vi "ReadAllChnlParams.vi"(8 "error in (no error)":errorcluster, 10 "ChnlName":string, 11 "BME_DG_System in":refnum<class "BME_DG_System.lvclass">) -> (0 "error out":errorcluster, 1 "Name of Card":string, 2 "ChnlParam":T1={"Channel Name"="", "ChnParameter"={" Delay (µs)"=0.0, "On?"=FALSE, "PositiveVoltage?"=TRUE, "50OhmTerminated? "=FALSE, "25OhmOutput?"=FALSE}, "DelayFormula"="", "OutputModulo"=1, "Go and Done Signal"={"Go Signal"=16, "Done Signal"=16}, "G08_Chnl_Settings"={"Pulse Width (µs)"=0.1, "Output Offset"=0, "Disconnect (E,F)"=FALSE, "Onto MsBus (E,F)"=FALSE, "Input Positive (E,F)"=TRUE, "Param Change"=FALSE, "Inhibit internal clock"=FALSE}} {"ChnParameter"."Delay (µs)" min=0.0 max=100000000.0 format="%.4f"; "G08_Chnl_Settings"."Pulse Width (µs)" min=0.0 max=8947840.0 format="%#.6f"; "Go and Done Signal"."Done Signal" format="%04x" items=["Local Primary"=1, "Local Secondary"=2, "Local Force"=4, "Master Primary"=16]; "Go and Done Signal"."Go Signal" format="%04x" items=["Local Primary0x1"=1, "Local Secondary0x2"=2, "Local Force 0x4"=4, "Resynchronize 0x8"=8, "Master Prim. 0x10"=16, "Master Sec. 0x20"=32, "Master Force  0x40"=64, "System Clock 0x80"=128, "Delay Clock 0x100"=256, "Inhibit Local 0x200"=512, "Start Local 0x400"=1024, "Start Bus 0x800"=2048, "Step Back Local 0x1000"=4096, "Step Back Bus 0x2000"=8192, "RunCircle 0x4000"=16384, "SyncReload 0x8000"=32768, "From E 0x10000"=65536, "From F 0x20000"=131072, "From Bus 0x40000"=262144]}, 3 "BME_DG_System out":refnum<class "BME_DG_System.lvclass">)   [LabVIEW 2009, in "POLARIS BME DG.lvlib" / "BME_DG_System.lvclass"]
uses:
  BME_DG_System.lvclass
  Chnl Settings Complete.ctl
  LV-BME Interface/ChnlSettings.ctl
  Go_Done_Chnl_Settings.ctl
  MSBus.ctl
  SG08_Chnl_Settings.ctl
  BME_DG_G08_Chnl/BME_DG_G08_Chnl.lvclass
  BME_DG_G05P2_Chnl/BME_DG_G05P2_Chnl.lvclass
  BME_DG_Chnl/BME_DG_Chnl.lvclass
  POLARIS BME DG.lvlib
  BME_DG_Base/BME_DG_Base.lvclass
panel:
  in  "ChnlParam 2":T1 {"ChnParameter"."Delay (µs)" min=0.0 max=100000000.0 format="%.4f"; "G08_Chnl_Settings"."Pulse Width (µs)" min=0.0 max=8947840.0 format="%#.6f"; "Go and Done Signal"."Done Signal" format="%04x" items=["Local Primary"=1, "Local Secondary"=2, "Local Force"=4, "Master Primary"=16]; "Go and Done Signal"."Go Signal" format="%04x" items=["Local Primary0x1"=1, "Local Secondary0x2"=2, "Local Force 0x4"=4, "Resynchronize 0x8"=8, "Master Prim. 0x10"=16, "Master Sec. 0x20"=32, "Master Force  0x40"=64, "System Clock 0x80"=128, "Delay Clock 0x100"=256, "Inhibit Local 0x200"=512, "Start Local 0x400"=1024, "Start Bus 0x800"=2048, "Step Back Local 0x1000"=4096, "Step Back Bus 0x2000"=8192, "RunCircle 0x4000"=16384, "SyncReload 0x8000"=32768, "From E 0x10000"=65536, "From F 0x20000"=131072, "From Bus 0x40000"=262144]}
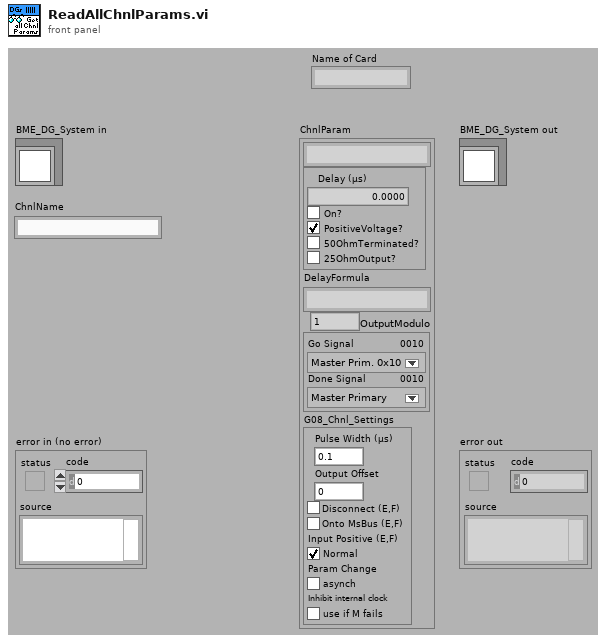
[diagram p1: front panel]
types:
  T1 = typedef "POLARIS BME DG.lvlib/Chnl Settings Complete.ctl" = cluster{"Channel Name":string, "ChnParameter":T2, "DelayFormula":string, "OutputModulo":i32, "Go and Done Signal":T3, "G08_Chnl_Settings":T5}
  T2 = typedef "POLARIS BME DG.lvlib/ChnlSettings.ctl" = cluster{" Delay (µs)":dbl, "On?":bool, "PositiveVoltage?":bool, "50OhmTerminated? ":bool, "25OhmOutput?":bool}
  T3 = typedef "POLARIS BME DG.lvlib/Go_Done_Chnl_Settings.ctl" = cluster{"Go Signal":T4, "Done Signal":u32}
  T4 = typedef "POLARIS BME DG.lvlib/MSBus.ctl" = u32
  T5 = typedef "POLARIS BME DG.lvlib/SG08_Chnl_Settings.ctl" = cluster{"Pulse Width (µs)":dbl, "Output Offset":u32, "Disconnect (E,F)":bool, "Onto MsBus (E,F)":bool, "Input Positive (E,F)":bool, "Param Change":bool, "Inhibit internal clock":bool}
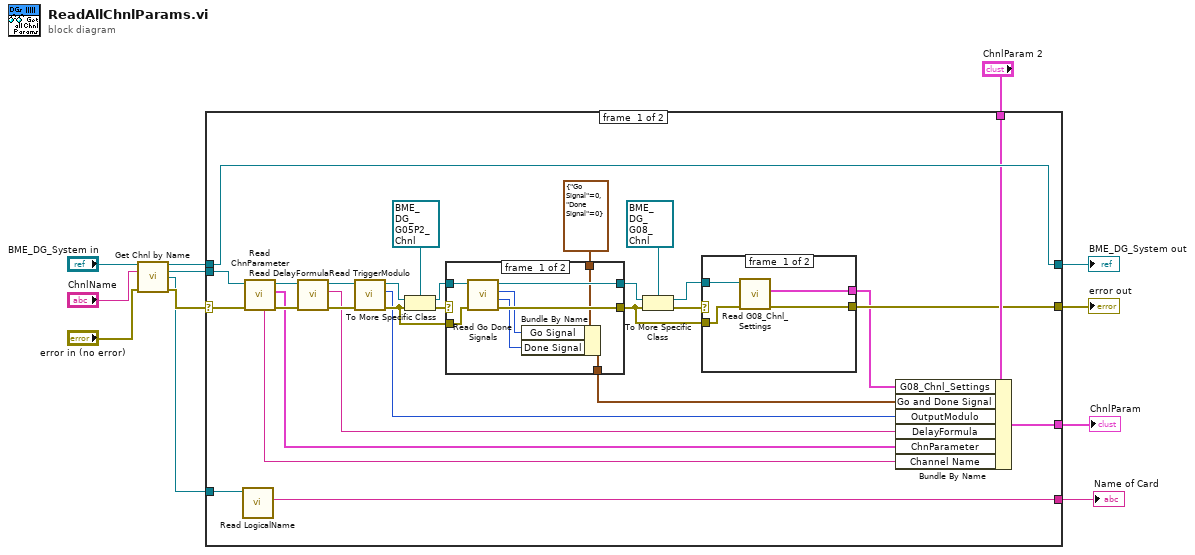
[diagram p0: block diagram]
diagram:
  n1 = call "Get Chnl by Name.vi"("BME_DG_System in"="BME_DG_System in", "Chnl Name"="ChnlName", "error in (no error)"="error in (no error)") -> ("BME_DG_System out"=w9:refnum<class "BME_DG_System.lvclass">, "BME_DG_Chnl"=w6:refnum<class "BME_DG_Chnl.lvclass">, "Owner DG"=w2:refnum<class "BME_DG_Base.lvclass">, "error out"=w7:errorcluster)  [unwired: 7 in, 2 out]
  n2 = case shown="No Error" w7 {
    selector: w7 -> [w38 w60]
    tunnel: [w23 w60] -> w12
    tunnel: [w41 w59] -> w11
    tunnel: w9 -> [w41 w59]
    tunnel: w6 -> [w39 _]
    tunnel: "ChnlParam 2" -> [w40 w58]
    tunnel: [w33 w58] -> w4
    tunnel: w2 -> [w14 _]
    tunnel: [w13 _] -> w1
    frame #0 {
      n3 = call "Read LogicalName.vi"("BME_DG_Base in"=w14) -> ("LogicalName"=w13:string)  [unwired: 8 in, 2 out]
      n4 = call-dynamic "Read ChnParameter.vi"("error in (no error)"=w38, "BME_DG_Chnl in"=w39) -> ("error out"=w36:errorcluster, "ChnParemater"=w18:T2, "BME_DG_Chnl out"=w37:refnum<class "BME_DG_Chnl.lvclass">, "Name"=w15:string)  [unwired: 4 in, 2 out]
      n5 = call-dynamic "Read DelayFormula.vi"("error in (no error)"=w36, "BME_DG_Chnl in"=w37) -> ("error out"=w34:errorcluster, "DelayFormula"=w17:string, "BME_DG_Chnl out"=w35:refnum<class "BME_DG_Chnl.lvclass">)  [unwired: 7 in]
      n6 = call-dynamic "Read TriggerModulo.vi"("error in (no error)"=w34, "BME_DG_Chnl in"=w35) -> ("error out"=w28:errorcluster, "TriggerModulo"=w16:i32, "BME_DG_Chnl out"=w32:refnum<class "BME_DG_Chnl.lvclass">)  [unwired: 7 in]
      n7 = To More Specific Class(target class=refnum<class "BME_DG_G05P2_Chnl.lvclass"> refnum ("POLARIS BME DG.lvlib:BME_DG_G05P2_Chnl.lvclass"), reference=w32, error in=w28) -> (specific class reference=w30:refnum<class "BME_DG_G05P2_Chnl.lvclass">, error out=w29:errorcluster)
      n8 = case shown="No Error" w29 {
        tunnel: w30 -> [w54 w56]
        tunnel: [w53 w57] -> w25
        tunnel: [w52 w56] -> w22
        tunnel: w28 -> [w47 w57]
        tunnel: T3 {"Go Signal"=0, "Done Signal"=0} ("Go and Done Signal") -> [w49 w55]
        tunnel: [w48 w55] -> w19
        frame #0 {
          n9 = call-dynamic "Read Go Done Signals.vi"("error in (no error)"=w47, "BME_DG_G05P2_Chnl in"=w54) -> ("error out"=w53:errorcluster, "Done Signal"=w50:u32, "Go Signal"=w51:u32, "BME_DG_G05P2_Chnl out"=w52:refnum<class "BME_DG_G05P2_Chnl.lvclass">)  [unwired: 6 in]
          n10 = Bundle By Name(cluster=w49, "Go Signal"=w51, "Done Signal"=w50) -> (w48:T3)
        }
        frame #1 {
        }
      }
      n11 = To More Specific Class(target class=refnum<class "BME_DG_G08_Chnl.lvclass"> refnum ("POLARIS BME DG.lvlib:BME_DG_G08_Chnl.lvclass"), reference=w22, error in=w25) -> (specific class reference=w24:refnum<class "BME_DG_G08_Chnl.lvclass">, error out=w26:errorcluster)
      n12 = case shown="No Error" w26 {
        tunnel: w25 -> [w44 w46]
        tunnel: w24 -> [w45 _]
        tunnel: [w43 w46] -> w23
        tunnel: [w42 _] -> w20
        frame #0 {
          n13 = call-dynamic "Read G08_Chnl_Settings.vi"("error in (no error)"=w44, "BME_DG_G08_Chnl in"=w45) -> ("error out"=w43:errorcluster, "G08_Chnl_Settings"=w42:T5)  [unwired: 7 in, 1 out]
        }
        frame #1 {
        }
      }
      n14 = Bundle By Name(cluster=w40, "G08_Chnl_Settings"=w20, "Go and Done Signal"=w19, "OutputModulo"=w16, "DelayFormula"=w17, "ChnParameter"=w18, "Channel Name"=w15) -> (w33:T1)
    }
    frame #1 {
    }
  }
  "error out" <- w12
  "BME_DG_System out" <- w11
  "ChnlParam" <- w4
  "Name of Card" <- w1
